vi "LINX PWM Benchmark.vi"() -> ()   [LabVIEW 2013]
uses:
  <vilib>/LabVIEW Hacker/LINX/Private/Type Defs/Peripherals/PWM/PWM Duty Cycle Control.ctl
  <vilib>/LabVIEW Hacker/LINX/Private/Type Defs/Interface.ctl
  <vilib>/LabVIEW Hacker/LINX/Private/Device/Device.lvlib
  <vilib>/LabVIEW Hacker/LINX/LVH-LINX.lvlib
  <vilib>/ptbypt/NI_PtbyPt.lvlib
panel:
  in  "Duty Cycles":T1[](array[typedef])
  out "Device Name":string
  in  "Stop Button":bool
  out "Loop Rate":dbl(graph)
  out "Loop Time (ms)":i32
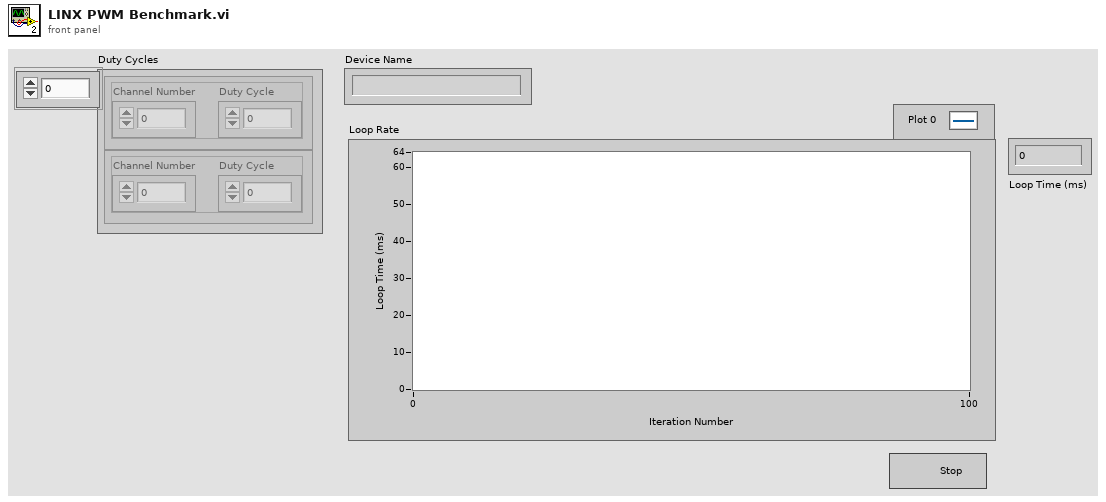
[diagram p1: front panel]
types:
  T1 = typedef "LVH-LINX.lvlib/PWM Duty Cycle Control.ctl" = cluster{"Channel Number":u8, "Duty Cycle":u8}
  T2 = typedef "LVH-LINX.lvlib/Interface.ctl" = enum16{"Serial", "TCP"}
  T3 = typedef "LVH-LINX.lvlib/Device.lvlib/LINX Device Config.ctl" = cluster{"Interface":T2, "COM Port":refnum<visa-resource-name>, "TCP Configuration":T4, "Device Family":T5, "Device ID":u8, "Device Name":string, "TCP Ref":refnum<k5>}
  T4 = typedef "LVH-LINX.lvlib/Device.lvlib/TCP Config.ctl" = cluster{"IP Address":string, "Port":u16}
  T5 = typedef "LVH-LINX.lvlib/Device Family.ctl" = enum8{"National Instruments", "Digilent", "Arduino"}
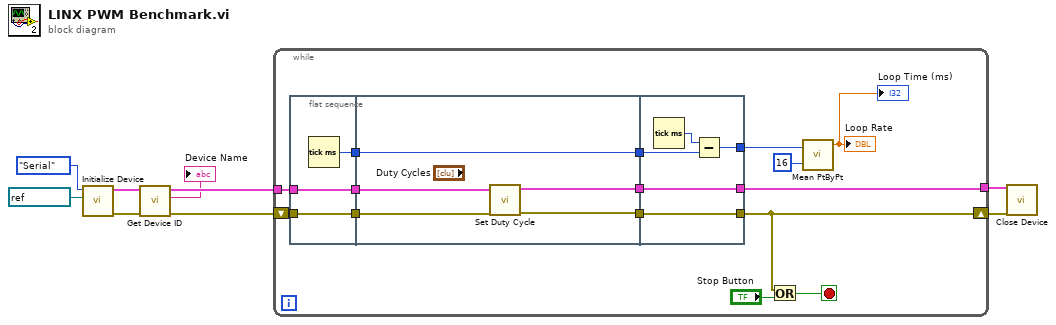
[diagram p0: block diagram]
diagram:
  n1 = call <vilib>:"Initialize Device.vi"("COM Port"=refnum<visa-resource-name> "COM5", "Interface"=Interface."Serial") -> ("Error Out"=w5:errorcluster, "LINX Device Config"=w6:T3)  [unwired: 7 in, 1 out]
  n2 = call <vilib>:"Get Device ID.vi"("Error In"=w5, "LINX Device Config"=w6) -> ("Error Out"=w4:errorcluster, "Device Name"=→"Device Name":string, "LINX Device Config"=w3:T3)  [unwired: 7 in]
  n3 = while {
    tunnel: w3 -> [w24]
    shift-right: [w10] -> w7
    shift-left: w4 -> [w12]
    tunnel: [w15] -> w1
    stop <- w23 stop-if-true
    n4 = flat-sequence {
      tunnel: w24 -> [w27]
      tunnel: [w27] -> w21
      tunnel: [w26] -> w20
      tunnel: w12 -> [w25]
      tunnel: [w25] -> w11
      tunnel: w21 -> [w30]
      tunnel: w20 -> [w32]
      tunnel: [w32] -> w19
      tunnel: [w31] -> w14
      tunnel: [w28] -> w13
      tunnel: w11 -> [w29]
      tunnel: w19 -> [w36]
      tunnel: [w35] -> w18
      tunnel: [w34] -> w15
      tunnel: w14 -> [w34]
      tunnel: w13 -> [w33]
      tunnel: [w33] -> w10
      frame #0 {
        n5 = Tick Count (ms)() -> (millisecond timer value=w26:u32)
      }
      frame #1 {
        n6 = call <vilib>:"Set Duty Cycle.vi"("Error In"=w29, "LINX Device Config"=w30) -> ("Error Out"=w28:errorcluster, "LINX Device Config"=w31:T3)  [unwired: 8 in]
      }
      frame #2 {
        n7 = Tick Count (ms)() -> (millisecond timer value=w37:u32)
        n8 = Subtract(x=w37, y=w36) -> (x-y=w35:u32)
      }
    }
    n9 = Or(x=w10, y="Stop Button") -> (x .or. y?=w23:bool)
    n10 = call <vilib>:"Mean PtByPt.vi"("x"=w18, "sample length"=16) -> ("mean"=→"Loop Rate" →"Loop Time (ms)":dbl)  [unwired: 2 in, 1 out]
  }
  n11 = call <vilib>:"Close Device.vi"("Error In"=w7, "LINX Device Config"=w1) -> ()  [unwired: 8 in, 2 out]
